vi "I32 to ZigZag.vi"(11 "sint32":i32) -> (3 "ZigZag I32":i32)   [LabVIEW 2020, in "LV-Proto.lvlib"]
uses:
  LV-Proto.lvlib
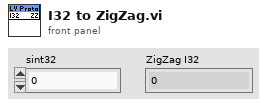
[diagram p1: front panel]
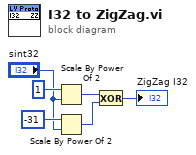
[diagram p0: block diagram]
diagram:
  n1 = Scale By Power Of 2(n=i16 1, x="sint32") -> (x*2^n=w3:i32)
  n2 = Scale By Power Of 2(n=i16 -31, x="sint32") -> (x*2^n=w2:i32)
  n3 = Exclusive Or(1:w2, 2:w3) -> (0:→"ZigZag I32":i32)
